vi "Send Last Ack.vi"(8 "error in (no error)":errorcluster, 10 "Message Transport Queue in":refnum<class "Message Transport Queue.lvclass">, 11 "Mediated Asynchronous Actor":refnum<class "Mediated Asynchronous Actor.lvclass">) -> (0 "error out":errorcluster)   [LabVIEW 2016, in "Stream Mediator.lvlib" / "Last Ack.lvclass"]
doc: "--\nCopyright © 2017 Composed SystemsI All rights reserved.\n\nAuthor: Jon McBee <jon.mcbee@composed.io>\n\nThis library is provided \"AS IS\" ,WITHOUT WARRANTIES OR\nCONDITIONS OF ANY KIND, either express or implied.\n\nComposed Systems -- composed.io\n\nStream 0.0.1.1\nJon McBee - Composed Systems\nCopyright (c) 2017, Composed Systems"
uses:
  <userlib>/Composed Systems/Stream/Mediator/Classes/Message Command Last Ack/Last Ack.lvclass
  <userlib>/Composed Systems/Stream/Mediator/Classes/Mediated Asynchronous Actor/Mediated Asynchronous Actor.lvclass
  <userlib>/Composed Systems/Stream/Mediator/Classes/Message Transport Queue/Message Transport Queue.lvclass
  <userlib>/Composed Systems/Stream/Mediator/Classes/Message Transport Interface/Message Priority.ctl
  C:/Program Files (x86)/National Instruments/LabVIEW 2016/user.lib/Composed Systems/Stream/Mediator/Classes/Message Interface/Message Interface.lvclass
  <userlib>/Composed Systems/Stream/Mediator/Classes/Message Command Last Ack/Last Ack.lvclass/Last Ack.ctl
  <userlib>/Composed Systems/Stream/Mediator/Classes/Message Transport Interface/Message Transport Interface.lvclass
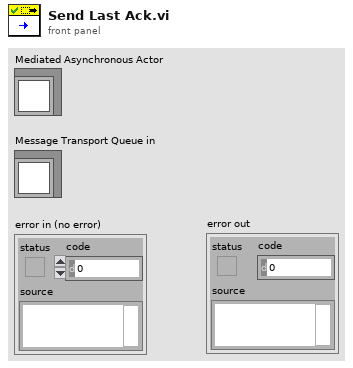
[diagram p1: front panel]
types:
  T1 = typedef "Stream Mediator.lvlib/Message Transport Interface.lvclass/Message Priority.ctl" = enum16{"Normal", "High"}
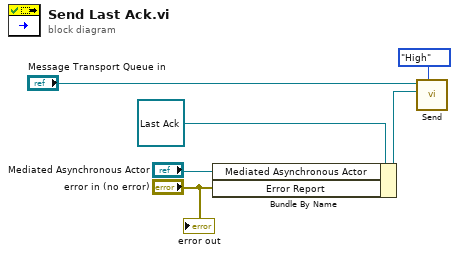
[diagram p0: block diagram]
diagram:
  n1 = Bundle By Name(cluster=refnum<class "Last Ack.lvclass"> refnum ("Mediator Framework.lvlib:Last Ack.lvclass"), "Mediated Asynchronous Actor"="Mediated Asynchronous Actor", "Error Report"="error in (no error)") -> (w1:refnum<class "Last Ack.lvclass">)
  n2 = call-dynamic "Send.vi"("Message Priority"=Message_Priority."High", "Message"=w1, "Message Transport Queue in"="Message Transport Queue in") -> ()  [unwired: 6 in, 3 out]
  "error out" <- "error in (no error)"
